vi "appendArray.vi"(8 "error in (no error)":errorcluster, 10 "ScriptEvent":refnum<class "ScriptEvent.lvclass">, 11 "ScriptEventList in":refnum<class "ScriptEventList.lvclass">) -> (0 "error out":errorcluster, 2 "size":i32, 3 "ScriptEventList out":refnum<class "ScriptEventList.lvclass">)   [LabVIEW 2009, in "Tools.lvlib" / "Scripting.lvlib" / "ScriptEventList.lvclass"]
uses:
  ScriptEventList.lvclass
  ScriptEvent.lvclass
  ScriptEventList.lvclass/ScriptEventList.ctl
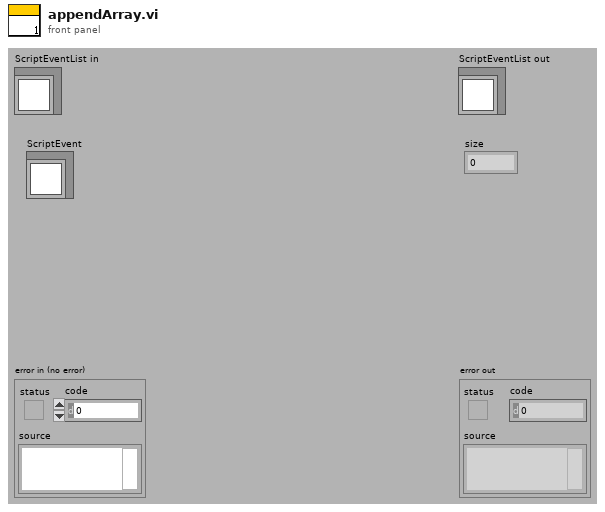
[diagram p1: front panel]
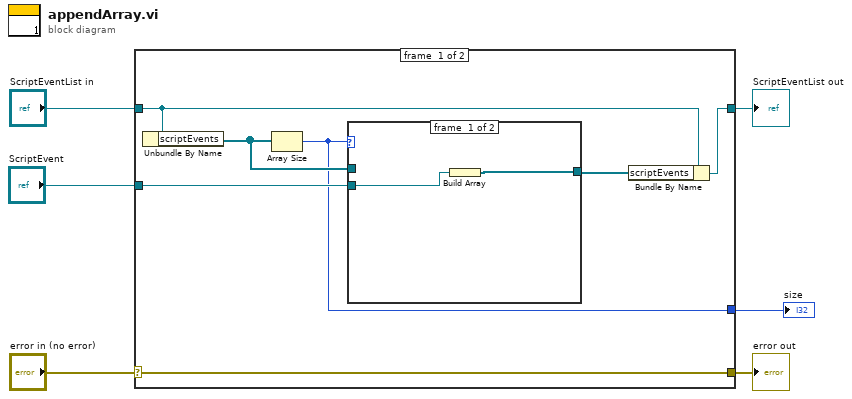
[diagram p0: block diagram]
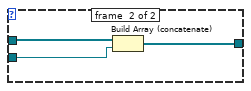
[diagram p2: hidden frame]
diagram:
  n1 = case shown="No Error" "error in (no error)" {
    selector: "error in (no error)" -> [w13 w20]
    tunnel: [w13 w20] -> w5
    tunnel: [w8 w19] -> w3
    tunnel: "ScriptEventList in" -> [w9 w19]
    tunnel: "ScriptEvent" -> [w11 _]
    tunnel: [w7 _] -> w1
    frame #0 {
      n2 = Unbundle By Name(w9) -> ("scriptEvents"=w12:refnum<class "ScriptEvent.lvclass">[])
      n3 = Array Size(array=w12) -> (size(s)=w7:i32)
      n4 = case shown="0" w7 {
        tunnel: w12 -> [_ w18]
        tunnel: w11 -> [w15 w17]
        tunnel: [w14 w16] -> w10
        frame #0 {
          n5 = Build Array(w15) -> (w14:refnum<class "ScriptEvent.lvclass">[])
        }
        frame #1 {
          n6 = Build Array (concatenate)(w18, w17) -> (w16:refnum<class "ScriptEvent.lvclass">[])
        }
      }
      n7 = Bundle By Name(cluster=w9, "scriptEvents"=w10) -> (w8:refnum<class "ScriptEventList.lvclass">)
    }
    frame #1 {
    }
  }
  "error out" <- w5
  "ScriptEventList out" <- w3
  "size" <- w1
